vi "ExcelForDispatch.vi"(8 "error out":errorcluster, 9 "RowNo":i32, 10 "array":variant[][](array[variant]), 11 "report out":refnum<class "NI_report.lvclass">) -> (0 "error out 2":errorcluster, 1 "Numeric":i32, 3 "report out 2":refnum<class "NI_report.lvclass">)   [LabVIEW 2012]
uses:
  <vilib>/Utility/NIReport.llb/NI_report.lvclass
  <vilib>/addons/database/_DB Variant To Data/Database Variant To Data.xnode
  <vilib>/Utility/NIReport.llb/Excel/NI_Excel.lvclass
panel:
  out "x+y":i32
  out "ExcelRow":i32
  in  "start (0, 0) 4":cluster{"start row":i32, "start column":i32}
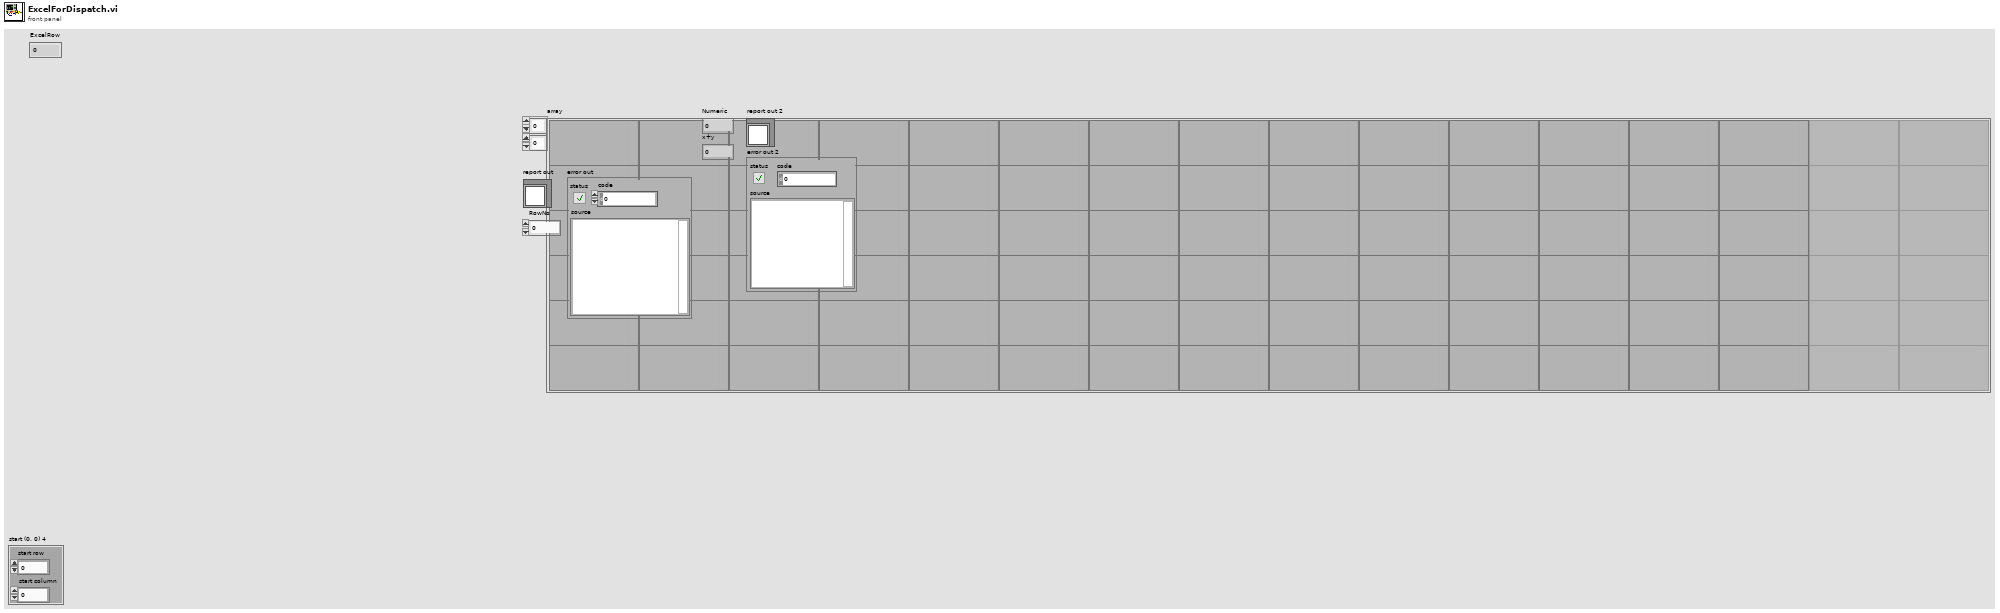
[diagram p1: front panel]
types:
  T1 = cluster{"on/off":bool, "weight":i32, "color":u32}
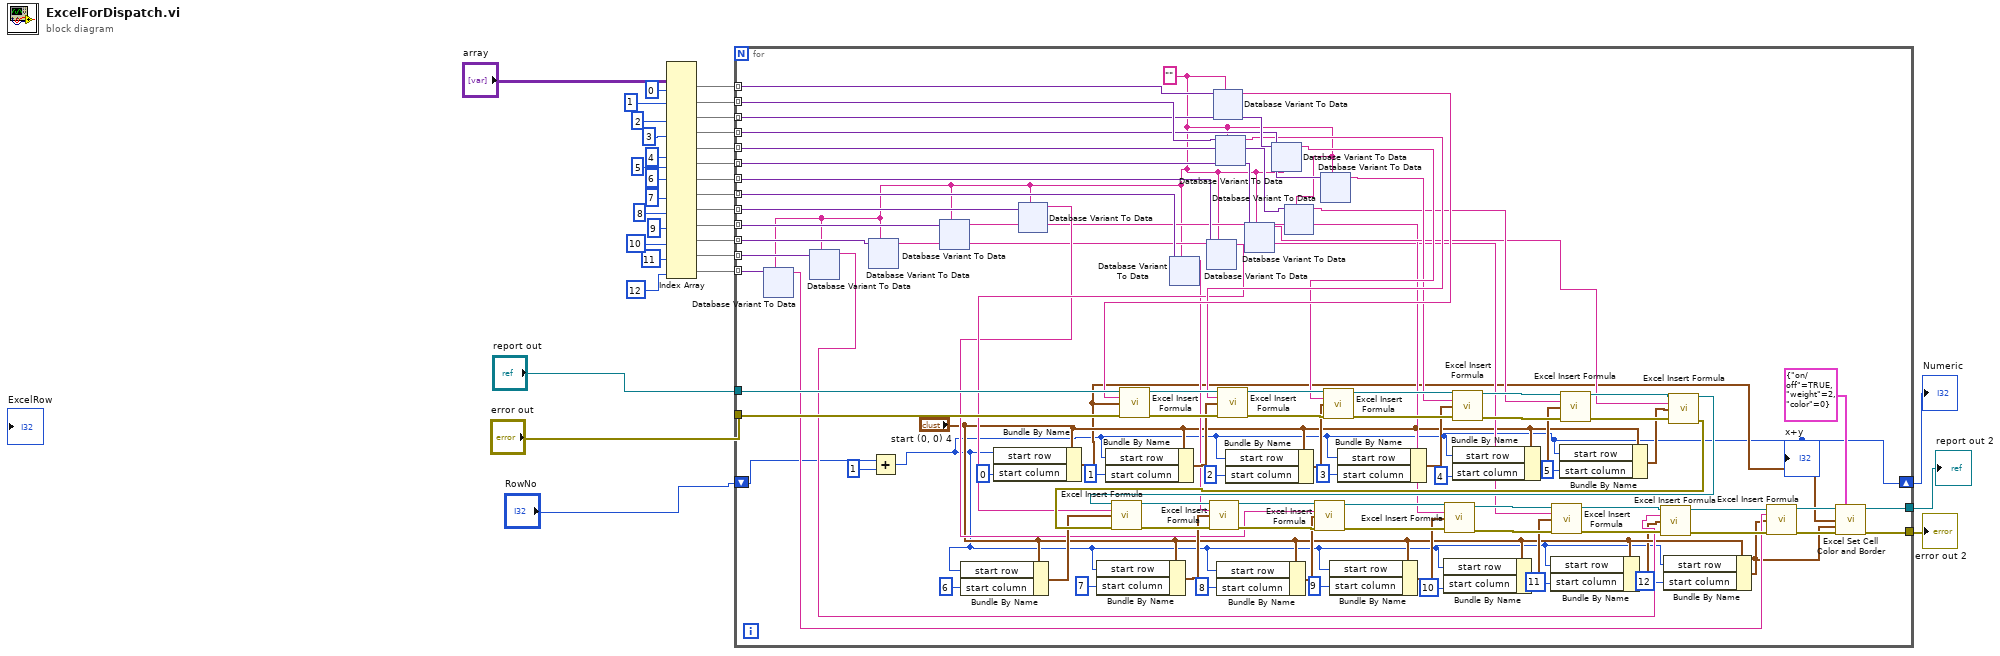
[diagram p0: block diagram]
diagram:
  n1 = Index Array(array="array", index (col) #1=0 ("disabled index (col)"), index (col) #2=1 ("index (col)"), index (col) #3=2 ("index (col)"), index (col) #4=3 ("index (col)"), index (col) #5=4 ("index (col)"), index (col) #6=5 ("index (col)"), index (col) #7=6 ("index (col)"), index (col) #8=7 ("index (col)"), index (col) #9=8 ("index (col)"), index (col) #10=9 ("index (col)"), index (col) #11=10 ("index (col)"), index (col) #12=11 ("index (col)"), index (col) #13=12 ("index (col)")) -> (element #1=w25:variant[], element #2=w24:variant[], element #3=w23:variant[], element #4=w22:variant[], element #5=w21:variant[], element #6=w20:variant[], element #7=w19:variant[], element #8=w18:variant[], element #9=w14:variant[], element #10=w13:variant[], element #11=w12:variant[], element #12=w10:variant[], element #13=w8:variant[])  [unwired: 13 in]
  n2 = for {
    tunnel: w25 -> [w121] mode=indexing
    tunnel: w24 -> [w120] mode=indexing
    tunnel: w23 -> [w119] mode=indexing
    tunnel: w22 -> [w118] mode=indexing
    tunnel: w21 -> [w117] mode=indexing
    tunnel: w20 -> [w116] mode=indexing
    tunnel: w19 -> [w115] mode=indexing
    tunnel: w18 -> [w114] mode=indexing
    tunnel: "report out" -> [w113]
    tunnel: "error out" -> [w112]
    tunnel: w14 -> [w59] mode=indexing
    tunnel: w13 -> [w58] mode=indexing
    tunnel: w12 -> [w57] mode=indexing
    tunnel: w10 -> [w53] mode=indexing
    tunnel: w8 -> [w51] mode=indexing
    tunnel: [w38] -> w4
    tunnel: [w37] -> w3
    shift-right: [w36] -> w2
    shift-left: "RowNo" -> [w35]
    w50 = ""
    n3 = xnode "Database Variant To Data"("database variant"=w51, "type"=w50) -> ("data"=w44:string)  [unwired: 1 in, 1 out]
    n4 = xnode "Database Variant To Data"("database variant"=w53, "type"=w50) -> ("data"=w52:string)  [unwired: 1 in, 1 out]
    n5 = xnode "Database Variant To Data"("database variant"=w57, "type"=w50) -> ("data"=w54:string)  [unwired: 1 in, 1 out]
    n6 = Add(x=w35, y=1) -> (x+y=w36:i32)
    "x+y" <- w36
    n7 = xnode "Database Variant To Data"("database variant"=w58, "type"=w50) -> ("data"=w55:string)  [unwired: 1 in, 1 out]
    n8 = Bundle By Name(cluster="start (0, 0) 4", "start row"=w36, "start column"=6) -> (w62:cluster{"start row":i32, "start column":i32})
    n9 = Bundle By Name(cluster="start (0, 0) 4", "start row"=w36, "start column"=0) -> (w40:cluster{"start row":i32, "start column":i32})
    n10 = xnode "Database Variant To Data"("database variant"=w59, "type"=w50) -> ("data"=w56:string)  [unwired: 1 in, 1 out]
    n11 = Bundle By Name(cluster="start (0, 0) 4", "start row"=w36, "start column"=7) -> (w81:cluster{"start row":i32, "start column":i32})
    n12 = Bundle By Name(cluster="start (0, 0) 4", "start row"=w36, "start column"=1) -> (w105:cluster{"start row":i32, "start column":i32})
    n13 = xnode "Database Variant To Data"("database variant"=w114, "type"=w50) -> ("data"=w60:string)  [unwired: 1 in, 1 out]
    n14 = xnode "Database Variant To Data"("database variant"=w115, "type"=w50) -> ("data"=w61:string)  [unwired: 1 in, 1 out]
    n15 = xnode "Database Variant To Data"("database variant"=w121, "type"=w50) -> ("data"=w111:string)  [unwired: 1 in, 1 out]
    n16 = call <vilib>:"Excel Insert Formula.vi"("report in"=w113, "formula"=w111, "start (0, 0)"=w40, "error in (no error)"=w112) -> ("report out"=w108:refnum<class "NI_report.lvclass">, "error out"=w107:errorcluster)  [unwired: 10 in]
    n17 = xnode "Database Variant To Data"("database variant"=w120, "type"=w50) -> ("data"=w106:string)  [unwired: 1 in, 1 out]
    n18 = Bundle By Name(cluster="start (0, 0) 4", "start row"=w36, "start column"=8) -> (w77:cluster{"start row":i32, "start column":i32})
    n19 = call <vilib>:"Excel Insert Formula.vi"("report in"=w108, "formula"=w106, "start (0, 0)"=w105, "error in (no error)"=w107) -> ("report out"=w103:refnum<class "NI_report.lvclass">, "error out"=w102:errorcluster)  [unwired: 10 in]
    n20 = Bundle By Name(cluster="start (0, 0) 4", "start row"=w36, "start column"=2) -> (w101:cluster{"start row":i32, "start column":i32})
    n21 = xnode "Database Variant To Data"("database variant"=w116, "type"=w50) -> ("data"=w85:string)  [unwired: 1 in, 1 out]
    n22 = xnode "Database Variant To Data"("database variant"=w119, "type"=w50) -> ("data"=w100:string)  [unwired: 1 in, 1 out]
    n23 = xnode "Database Variant To Data"("database variant"=w117, "type"=w50) -> ("data"=w90:string)  [unwired: 1 in, 1 out]
    n24 = xnode "Database Variant To Data"("database variant"=w118, "type"=w50) -> ("data"=w95:string)  [unwired: 1 in, 1 out]
    n25 = call <vilib>:"Excel Insert Formula.vi"("report in"=w103, "formula"=w100, "start (0, 0)"=w101, "error in (no error)"=w102) -> ("report out"=w98:refnum<class "NI_report.lvclass">, "error out"=w97:errorcluster)  [unwired: 10 in]
    n26 = Bundle By Name(cluster="start (0, 0) 4", "start row"=w36, "start column"=9) -> (w73:cluster{"start row":i32, "start column":i32})
    n27 = Bundle By Name(cluster="start (0, 0) 4", "start row"=w36, "start column"=3) -> (w96:cluster{"start row":i32, "start column":i32})
    n28 = Bundle By Name(cluster="start (0, 0) 4", "start row"=w36, "start column"=10) -> (w69:cluster{"start row":i32, "start column":i32})
    n29 = Bundle By Name(cluster="start (0, 0) 4", "start row"=w36, "start column"=4) -> (w91:cluster{"start row":i32, "start column":i32})
    n30 = call <vilib>:"Excel Insert Formula.vi"("report in"=w98, "formula"=w95, "start (0, 0)"=w96, "error in (no error)"=w97) -> ("report out"=w93:refnum<class "NI_report.lvclass">, "error out"=w92:errorcluster)  [unwired: 10 in]
    n31 = Bundle By Name(cluster="start (0, 0) 4", "start row"=w36, "start column"=11) -> (w48:cluster{"start row":i32, "start column":i32})
    n32 = Bundle By Name(cluster="start (0, 0) 4", "start row"=w36, "start column"=5) -> (w86:cluster{"start row":i32, "start column":i32})
    n33 = call <vilib>:"Excel Insert Formula.vi"("report in"=w93, "formula"=w90, "start (0, 0)"=w91, "error in (no error)"=w92) -> ("report out"=w88:refnum<class "NI_report.lvclass">, "error out"=w87:errorcluster)  [unwired: 10 in]
    n34 = Bundle By Name(cluster="start (0, 0) 4", "start row"=w36, "start column"=12) -> (w39:cluster{"start row":i32, "start column":i32})
    n35 = call <vilib>:"Excel Insert Formula.vi"("report in"=w88, "formula"=w85, "start (0, 0)"=w86, "error in (no error)"=w87) -> ("report out"=w65:refnum<class "NI_report.lvclass">, "error out"=w64:errorcluster)  [unwired: 10 in]
    n36 = call <vilib>:"Excel Insert Formula.vi"("report in"=w65, "formula"=w61, "start (0, 0)"=w62, "error in (no error)"=w64) -> ("report out"=w83:refnum<class "NI_report.lvclass">, "error out"=w82:errorcluster)  [unwired: 10 in]
    n37 = call <vilib>:"Excel Insert Formula.vi"("report in"=w83, "formula"=w60, "start (0, 0)"=w81, "error in (no error)"=w82) -> ("report out"=w79:refnum<class "NI_report.lvclass">, "error out"=w78:errorcluster)  [unwired: 10 in]
    n38 = call <vilib>:"Excel Insert Formula.vi"("report in"=w79, "formula"=w56, "start (0, 0)"=w77, "error in (no error)"=w78) -> ("report out"=w75:refnum<class "NI_report.lvclass">, "error out"=w74:errorcluster)  [unwired: 10 in]
    n39 = call <vilib>:"Excel Insert Formula.vi"("report in"=w75, "formula"=w55, "start (0, 0)"=w73, "error in (no error)"=w74) -> ("report out"=w71:refnum<class "NI_report.lvclass">, "error out"=w70:errorcluster)  [unwired: 10 in]
    n40 = call <vilib>:"Excel Insert Formula.vi"("report in"=w71, "formula"=w54, "start (0, 0)"=w69, "error in (no error)"=w70) -> ("report out"=w67:refnum<class "NI_report.lvclass">, "error out"=w66:errorcluster)  [unwired: 10 in]
    n41 = call <vilib>:"Excel Insert Formula.vi"("report in"=w67, "formula"=w52, "start (0, 0)"=w48, "error in (no error)"=w66) -> ("report out"=w45:refnum<class "NI_report.lvclass">, "error out"=w46:errorcluster)  [unwired: 10 in]
    n42 = call <vilib>:"Excel Insert Formula.vi"("report in"=w45, "formula"=w44, "start (0, 0)"=w39, "error in (no error)"=w46) -> ("report out"=w43:refnum<class "NI_report.lvclass">, "error out"=w42:errorcluster)  [unwired: 10 in]
    n43 = call <vilib>:"Excel Set Cell Color and Border.vi"("report in"=w43, "inside border"=T1 {"on/off"=TRUE, "weight"=2, "color"=0}, "start (-1, -1)"=w40, "end (-1, -1)"=w39, "error in (no error)"=w42) -> ("report out"=w38:refnum<class "NI_report.lvclass">, "error out"=w37:errorcluster)  [unwired: 9 in]
  }
  "report out 2" <- w4
  "error out 2" <- w3
  "Numeric" <- w2
